vi "DestroyStationReferences.vi"() -> ()   [LabVIEW 2018]
uses:
  <vilib>/Instr/_visa.llb/VISA GPIB Control REN Mode.ctl
  Station References Global.vi
panel:
  in  "error in":errorcluster
  out "Error (ary)":errorcluster[](array[cluster])
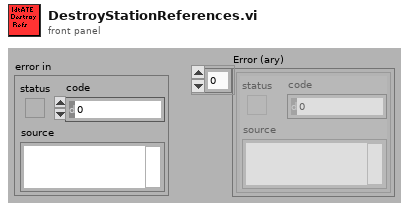
[diagram p1: front panel]
types:
  T1 = typedef "VISA GPIB Control REN Mode.ctl" = u16
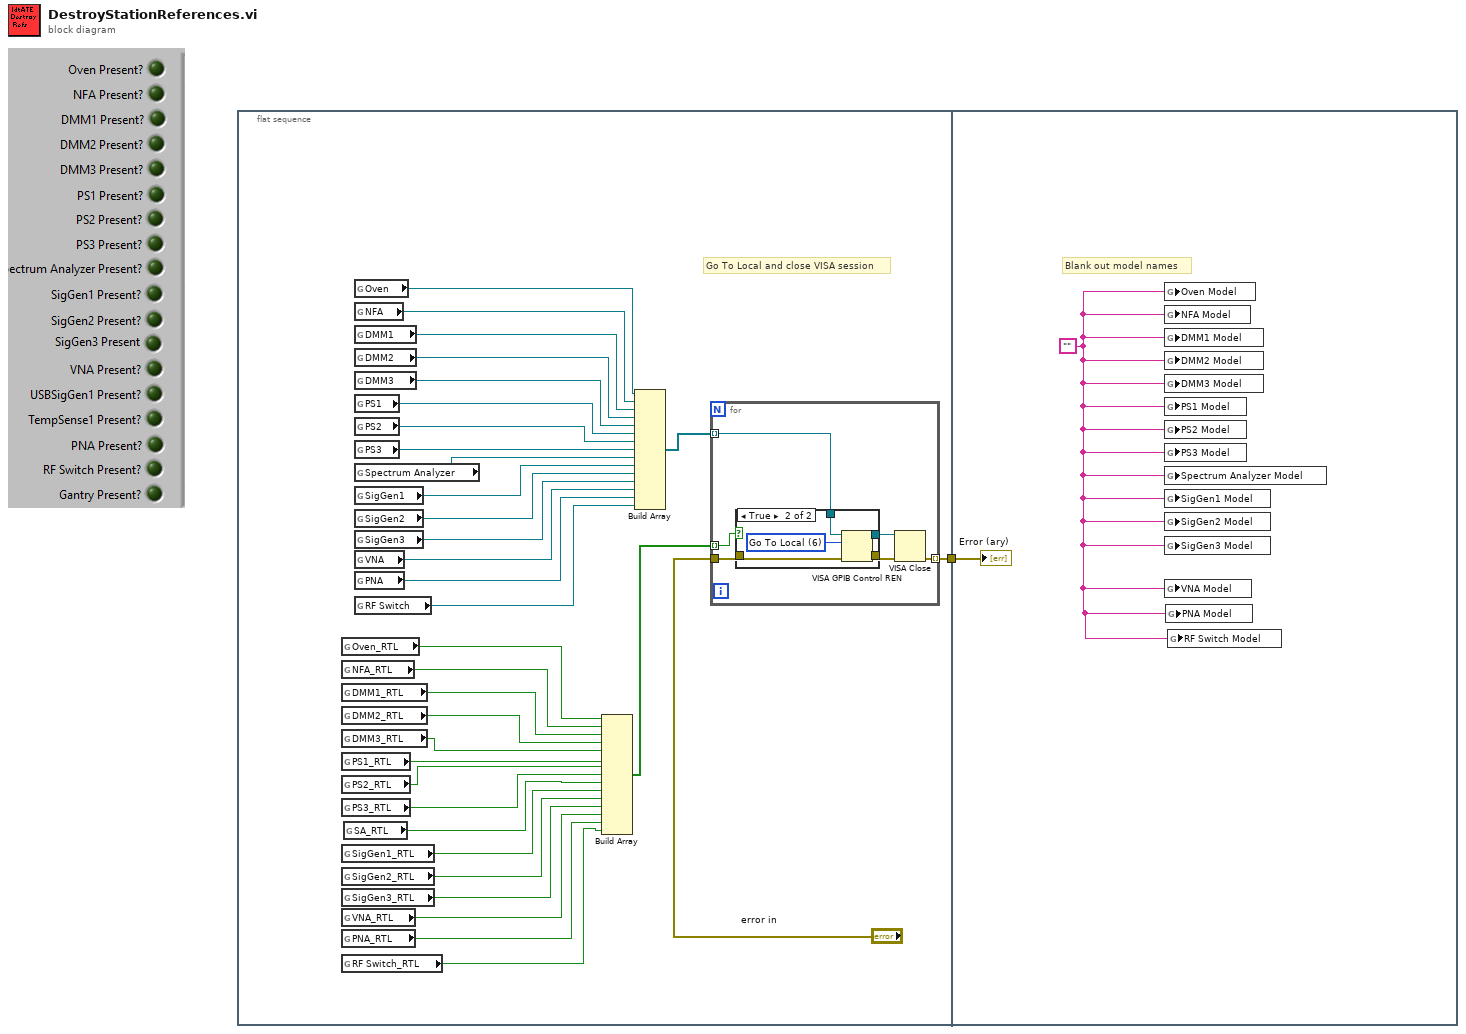
[diagram p0: block diagram]
diagram:
  n1 = flat-sequence {
    tunnel: [w33] -> w1
    tunnel: w1 -> [w50]
    frame #0 {
      # "Go To Local and close VISA session"
      n2 = global read "Station References Global.vi" "Oven_RTL"() -> (w17:bool)
      n3 = global read "Station References Global.vi" "NFA_RTL"() -> (w16:bool)
      n4 = global read "Station References Global.vi" "DMM1_RTL"() -> (w15:bool)
      n5 = global read "Station References Global.vi" "DMM2_RTL"() -> (w14:bool)
      n6 = global read "Station References Global.vi" "DMM3_RTL"() -> (w13:bool)
      n7 = global read "Station References Global.vi" "PS1_RTL"() -> (w12:bool)
      n8 = global read "Station References Global.vi" "PS2_RTL"() -> (w11:bool)
      n9 = global read "Station References Global.vi" "PS3_RTL"() -> (w10:bool)
      n10 = global read "Station References Global.vi" "SigGen1_RTL"() -> (w8:bool)
      n11 = global read "Station References Global.vi" "SigGen2_RTL"() -> (w7:bool)
      n12 = global read "Station References Global.vi" "SigGen3_RTL"() -> (w6:bool)
      n13 = global read "Station References Global.vi" "VNA_RTL"() -> (w5:bool)
      n14 = global read "Station References Global.vi" "PNA_RTL"() -> (w4:bool)
      n15 = global read "Station References Global.vi" "RF Switch_RTL"() -> (w3:bool)
      n16 = global read "Station References Global.vi" "SA_RTL"() -> (w9:bool)
      n17 = global read "Station References Global.vi" "Oven"() -> (w31:refnum<visa-resource-name>)
      n18 = global read "Station References Global.vi" "NFA"() -> (w30:refnum<visa-resource-name>)
      n19 = global read "Station References Global.vi" "DMM1"() -> (w29:refnum<visa-resource-name>)
      n20 = global read "Station References Global.vi" "DMM2"() -> (w28:refnum<visa-resource-name>)
      n21 = global read "Station References Global.vi" "DMM3"() -> (w27:refnum<visa-resource-name>)
      n22 = global read "Station References Global.vi" "PS1"() -> (w26:refnum<visa-resource-name>)
      n23 = global read "Station References Global.vi" "PS2"() -> (w25:refnum<visa-resource-name>)
      n24 = global read "Station References Global.vi" "PS3"() -> (w24:refnum<visa-resource-name>)
      n25 = global read "Station References Global.vi" "Spectrum Analyzer"() -> (w23:refnum<visa-resource-name>)
      n26 = global read "Station References Global.vi" "SigGen1"() -> (w22:refnum<visa-resource-name>)
      n27 = global read "Station References Global.vi" "SigGen2"() -> (w32:refnum<visa-resource-name>)
      n28 = global read "Station References Global.vi" "SigGen3"() -> (w21:refnum<visa-resource-name>)
      n29 = global read "Station References Global.vi" "VNA"() -> (w20:refnum<visa-resource-name>)
      n30 = global read "Station References Global.vi" "PNA"() -> (w19:refnum<visa-resource-name>)
      n31 = global read "Station References Global.vi" "RF Switch"() -> (w18:refnum<visa-resource-name>)
      n32 = Build Array(w17, w16, w15, w14, w13, w12, w11, w10, w9, w8, w7, w6, w5, w4, w3) -> (w2:bool[])
      n33 = Build Array(w31, w30, w29, w28, w27, w26, w25, w24, w23, w22, w32, w21, w20, w19, w18) -> (w34:refnum<visa-resource-name>[])
      n34 = for {
        tunnel: "error in" -> [w40]
        tunnel: w34 -> [w41] mode=indexing
        tunnel: [w37] -> w33 mode=indexing
        tunnel: w2 -> [w36] mode=indexing
        n35 = case shown="True" w36 {
          tunnel: w41 -> [w43 w48]
          tunnel: w40 -> [w42 w46]
          tunnel: [w43 w45] -> w39
          tunnel: [w42 w44] -> w38
          frame False {
          }
          frame True {
            w47 = T1 6 items=["Deassert REN", "Assert REN", "Go To Local; Deassert REN ", "Assert REN; Address Device", "Local Lockout (Addressed Devices)", "Local Lockout (This Device)", "Go To Local"] ("Mode")
            n36 = VISA GPIB Control REN(8:w46, 10:w47, 11:w48) -> (0:w44:errorcluster, 3:w45:refnum<visa-resource-name>)
          }
        }
        n37 = VISA Close(VISA resource name=w39, error in (no error)=w38) -> (error out=w37:errorcluster)
      }
    }
    frame #1 {
      w49 = ""
      # "Blank out model names"
      n38 = global write "Station References Global.vi" "Oven Model"(w49) -> ()
      n39 = global write "Station References Global.vi" "NFA Model"(w49) -> ()
      n40 = global write "Station References Global.vi" "DMM1 Model"(w49) -> ()
      n41 = global write "Station References Global.vi" "DMM2 Model"(w49) -> ()
      n42 = global write "Station References Global.vi" "DMM3 Model"(w49) -> ()
      n43 = global write "Station References Global.vi" "PS1 Model"(w49) -> ()
      n44 = global write "Station References Global.vi" "PS2 Model"(w49) -> ()
      n45 = global write "Station References Global.vi" "PS3 Model"(w49) -> ()
      n46 = global write "Station References Global.vi" "Spectrum Analyzer Model"(w49) -> ()
      n47 = global write "Station References Global.vi" "SigGen1 Model"(w49) -> ()
      n48 = global write "Station References Global.vi" "SigGen2 Model"(w49) -> ()
      n49 = global write "Station References Global.vi" "SigGen3 Model"(w49) -> ()
      n50 = global write "Station References Global.vi" "VNA Model"(w49) -> ()
      n51 = global write "Station References Global.vi" "PNA Model"(w49) -> ()
      n52 = global write "Station References Global.vi" "RF Switch Model"(w49) -> ()
      "Error (ary)" <- w50
    }
  }
